vi "Read Config File.vi"(11 "error in (no error)":errorcluster) -> (4 "Data Folder Path":path, 6 "Legend out":cluster{"Color Box":u32, "String":string}[](array[cluster]), 10 "Config File Sort":string, 15 "error out":errorcluster)   [LabVIEW 2018]
uses:
  <vilib>/Utility/config.llb/Read Key (Path).vi
  <vilib>/Utility/config.llb/Read Key (String).vi
  <vilib>/Utility/config.llb/Read Key (U32).vi
  <vilib>/Utility/config.llb/Write Key (String).vi
  <vilib>/Utility/config.llb/Write Key (Path).vi
  <vilib>/Utility/config.llb/Write Key (U32).vi
  <vilib>/Utility/config.llb/NI_LVConfig.lvlib
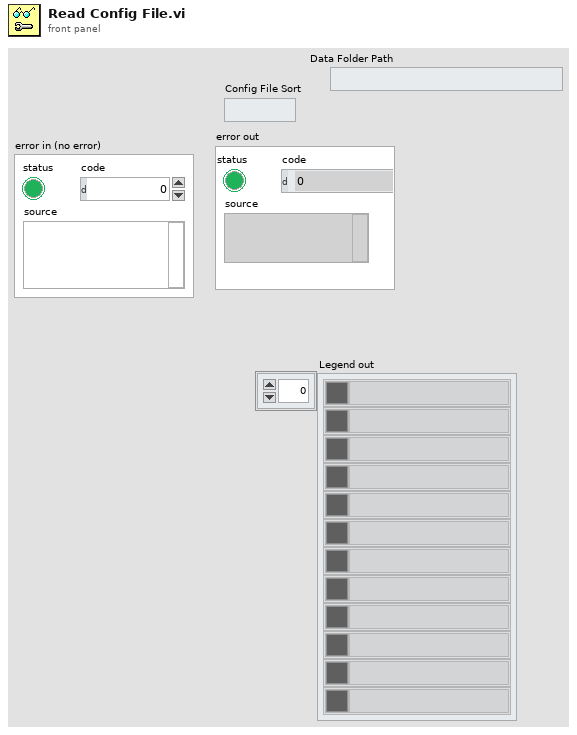
[diagram p1: front panel]
types:
  T1 = typedef "NI_LVConfig.lvlib/Config Data RefNum.ctl" = refnum<k1>
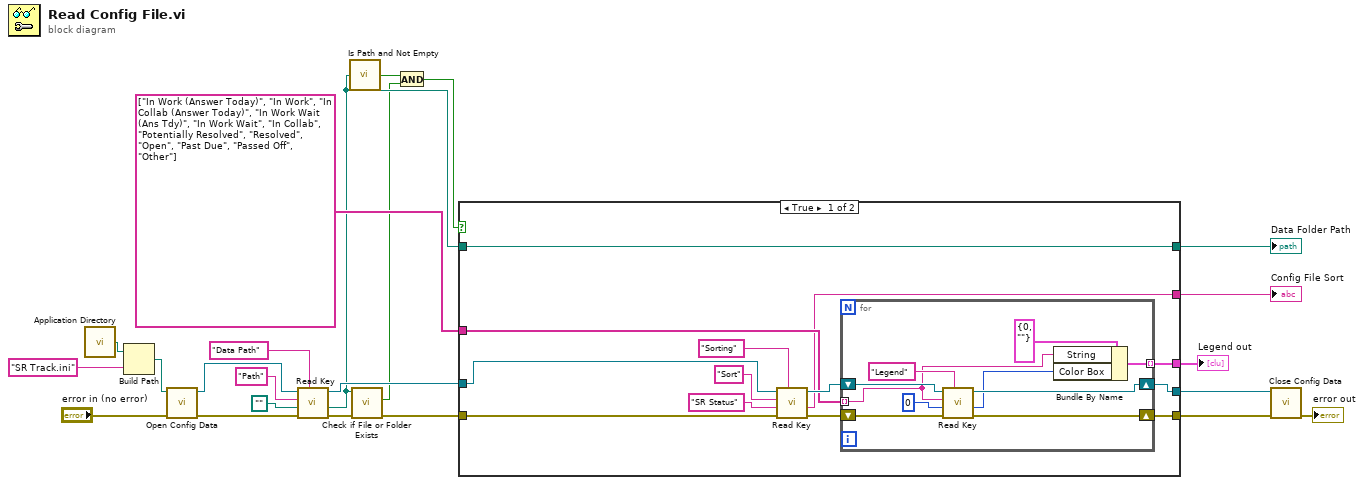
[diagram p0: block diagram]
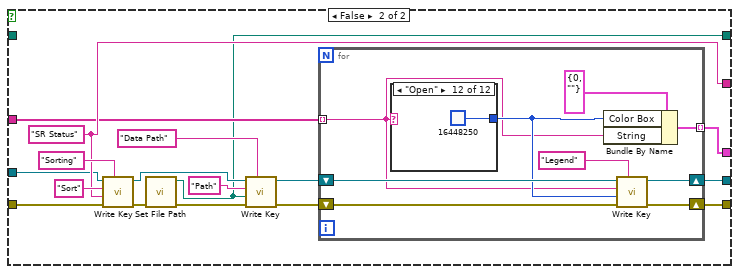
[diagram p2: hidden frame]
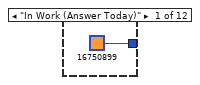
[diagram p3: hidden frame]
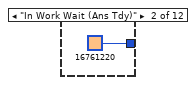
[diagram p4: hidden frame]
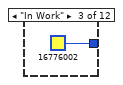
[diagram p5: hidden frame]
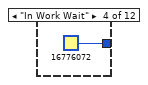
[diagram p6: hidden frame]
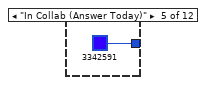
[diagram p7: hidden frame]
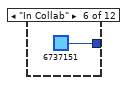
[diagram p8: hidden frame]
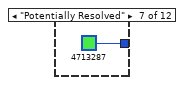
[diagram p9: hidden frame]
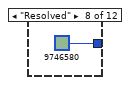
[diagram p10: hidden frame]
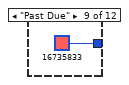
[diagram p11: hidden frame]
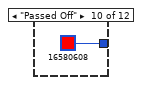
[diagram p12: hidden frame]
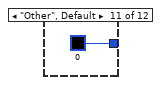
[diagram p13: hidden frame]
diagram:
  n1 = call <vilib>:"Application Directory.vi"() -> ("Application Directory"=w16:path)
  n2 = Build Path(base path=w16, name or relative path="SR Track.ini") -> (appended path=w20:path)
  n3 = call <vilib>:"Open Config Data.vi"("error in (no error)"="error in (no error)", "configuration file path"=w20) -> ("error out"=w12:errorcluster, "refnum"=w13:T1)  [unwired: 7 in, 1 out]
  n4 = call-poly <vilib>:"Read Key.vi"("section"="Data Path", "error in (no error)"=w12, "default value"=path "", "key"="Path", "refnum"=w13) -> ("error out"=w6:errorcluster, "value"=w5:path, "refnum out"=w11:T1)  [unwired: 3 in, 1 out]
  n5 = call <vilib>:"Is Path and Not Empty.vi"("path"=w5) -> ("Is Path and Not Empty?"=w3:bool)  [unwired: 4 in]
  n6 = call <vilib>:"Check if File or Folder Exists.vi"("error in (no error)"=w6, "path"=w5) -> ("error out"=w4:errorcluster, "file or folder exists?"=w2:bool)  [unwired: 7 in, 1 out]
  n7 = And(x=w3, y=w2) -> (x .and. y?=w1:bool)
  n8 = case shown="True" w1 {
    tunnel: [w32 w60] -> w21
    tunnel: [w25 w47] -> w8
    tunnel: [w24 w48] -> w9
    tunnel: string[] ["In Work (Answer Today)", "In Work", "In Collab (Answer Today)", "In Work Wait (Ans Tdy)", "In Work Wait", "In Collab", "Potentially Resolved", "Resolved", "Open", "Past Due", "Passed Off", "Other"] -> [w33 w59]
    tunnel: [w26 w62] -> w19
    tunnel: w11 -> [w27 w57]
    tunnel: w4 -> [w29 w58]
    tunnel: [w30 w49] -> w10
    tunnel: w5 -> [w30 _]
    frame True {
      n9 = call-poly <vilib>:"Read Key.vi"("section"="Sorting", "error in (no error)"=w29, "default value"="SR Status" ("key"), "key"="Sort", "refnum"=w27) -> ("error out"=w34:errorcluster, "value"=w32:string, "refnum out"=w35:T1)  [unwired: 3 in, 1 out]
      n10 = for {
        shift-right: [w46] -> w25
        shift-left: w35 -> [w44]
        shift-right: [w42] -> w24
        shift-left: w34 -> [w43]
        tunnel: w33 -> [w39] mode=indexing
        tunnel: [w40] -> w26 mode=indexing
        n11 = call-poly <vilib>:"Read Key.vi"("section"="Legend", "error in (no error)"=w43, "default value"=u32 0, "key"=w39, "refnum"=w44) -> ("error out"=w42:errorcluster, "value"=w38:u32, "refnum out"=w46:T1)  [unwired: 3 in, 1 out]
        n12 = Bundle By Name(cluster=cluster{"Color Box":u32, "String":string} {"Color Box"=0, "String"=""} ("element"), "String"=w39, "Color Box"=w38) -> (w40:cluster{"Color Box":u32, "String":string})
      }
    }
    frame False {
      w60 = "SR Status" ("key")
      n13 = call-poly <vilib>:"Write Key.vi"("section"="Sorting", "error in (no error)"=w58, "value"=w60, "key"="Sort", "refnum"=w57) -> ("error out"=w55:errorcluster, "refnum out"=w51:T1)  [unwired: 4 in, 1 out]
      n14 = call "Set File Path.vi"("error in"=w55) -> ("error out"=w56:errorcluster, "path"=w49:path)  [unwired: 9 in]
      n15 = call-poly <vilib>:"Write Key.vi"("section"="Data Path", "error in (no error)"=w56, "value"=w49, "key"="Path", "refnum"=w51) -> ("error out"=w54:errorcluster, "refnum out"=w53:T1)  [unwired: 4 in, 1 out]
      n16 = for {
        shift-right: [w72] -> w47
        shift-left: w53 -> [w70]
        shift-right: [w68] -> w48
        shift-left: w54 -> [w69]
        tunnel: w59 -> [w64] mode=indexing
        tunnel: [w65] -> w62 mode=indexing
        n17 = case shown="\"Open\"" w64 {
          tunnel: [u32 16750899 u32 16761220 u32 16776002 u32 16776072 u32 3342591 u32 6737151 u32 4713287 u32 9746580 u32 16735833 u32 16580608 u32 0 u32 16448250] -> w66
          frame "In Work (Answer Today)" {
          }
          frame "In Work Wait (Ans Tdy)" {
          }
          frame "In Work" {
          }
          frame "In Work Wait" {
          }
          frame "In Collab (Answer Today)" {
          }
          frame "In Collab" {
          }
          frame "Potentially Resolved" {
          }
          frame "Resolved" {
          }
          frame "Past Due" {
          }
          frame "Passed Off" {
          }
          frame "Other", Default {
          }
          frame "Open" {
          }
        }
        n18 = Bundle By Name(cluster=cluster{"Color Box":u32, "String":string} {"Color Box"=0, "String"=""} ("element"), "Color Box"=w66, "String"=w64) -> (w65:cluster{"Color Box":u32, "String":string})
        n19 = call-poly <vilib>:"Write Key.vi"("section"="Legend", "error in (no error)"=w69, "value"=w66, "key"=w64, "refnum"=w70) -> ("error out"=w68:errorcluster, "refnum out"=w72:T1)  [unwired: 4 in, 1 out]
      }
    }
  }
  "Config File Sort" <- w21
  "Legend out" <- w19
  "Data Folder Path" <- w10
  n20 = call <vilib>:"Close Config Data.vi"("error in (no error)"=w9, "refnum"=w8) -> ("error out"=→"error out":errorcluster)  [unwired: 8 in, 1 out]
